vi "test_compressor.vi"() -> ()   [LabVIEW 2010]
panel:
  out "elapsed time":dbl[](array[numeric])
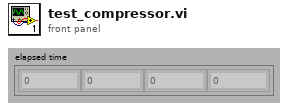
[diagram p1: front panel]
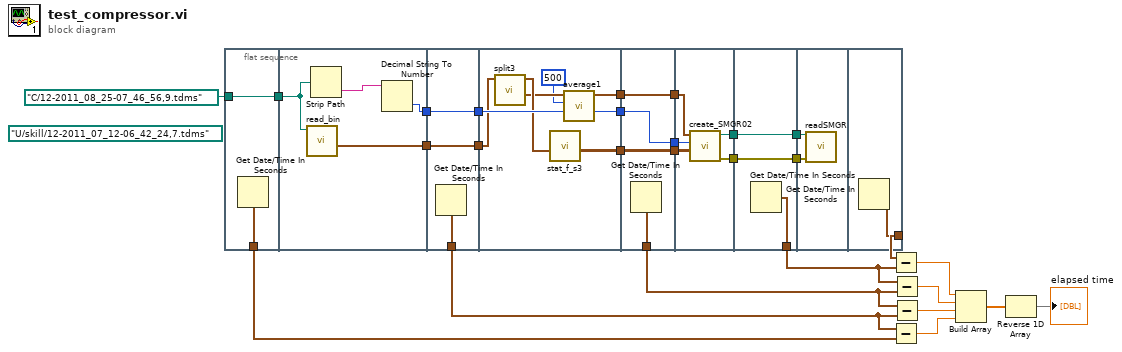
[diagram p0: block diagram]
diagram:
  (unwired) path "U:/skill/12-2011_07_12-06_42_24,7.tdms" ("datalog path (use dialog)")
  n1 = flat-sequence {
    tunnel: path "C:/12-2011_08_25-07_46_56,9.tdms" ("datalog path (use dialog)") -> [w29]
    tunnel: [w29] -> w26
    tunnel: [w28] -> w12
    tunnel: w26 -> [w32]
    tunnel: [w30] -> w24
    tunnel: [w31] -> w17
    tunnel: [w36] -> w25
    tunnel: w24 -> [w36]
    tunnel: w17 -> [w35]
    tunnel: [w35] -> w16
    tunnel: [w34] -> w9
    tunnel: w25 -> [w41]
    tunnel: [w43] -> w23
    tunnel: w16 -> [w42]
    tunnel: [w42] -> w15
    tunnel: [w38] -> w1
    tunnel: w23 -> [w47]
    tunnel: [w47] -> w22
    tunnel: w15 -> [w46]
    tunnel: [w46] -> w14
    tunnel: [w45] -> w10
    tunnel: [w44] -> w2
    tunnel: w1 -> [w44]
    tunnel: w22 -> [w52]
    tunnel: [w51] -> w20
    tunnel: [w50] -> w18
    tunnel: w14 -> [w49]
    tunnel: w2 -> [w48]
    tunnel: [w55] -> w21
    tunnel: w20 -> [w55]
    tunnel: [w54] -> w19
    tunnel: w18 -> [w54]
    tunnel: [w53] -> w11
    tunnel: w21 -> [w57]
    tunnel: w19 -> [w56]
    tunnel: [w58] -> w13
    frame #0 {
      n2 = Get Date/Time In Seconds() -> (seconds since 1Jan1904=w28:timestamp)
    }
    frame #1 {
      n3 = call "read_bin.vi"("datalog path"=w32) -> ("Waveform Graph"=w30:waveform(i16)[])  [unwired: 3 in, 3 out]
      n4 = Strip Path(path=w32) -> (name=w33:string)  [unwired: 1 out]
      n5 = Decimal String To Number(string=w33) -> (number=w31:i32)  [unwired: 2 in, 1 out]
    }
    frame #2 {
      n6 = Get Date/Time In Seconds() -> (seconds since 1Jan1904=w34:timestamp)
    }
    frame #3 {
      n7 = call "split3.vi"("Array of Waveform In"=w41) -> ("Sync"=w39:waveform(i16), "Array of Waveform"=w40:waveform(i16)[])  [unwired: 5 in]
      n8 = call "stat_f_s3.vi"("Array of Wfm"=w40) -> ("Array 2"=w43:waveform(i16)[][])  [unwired: 6 in]
      n9 = call "average1.vi"("Size"=500, "SignalIn"=w39) -> ("output waveform"=w38:waveform(i16))  [unwired: 5 in]
    }
    frame #4 {
      n10 = Get Date/Time In Seconds() -> (seconds since 1Jan1904=w45:timestamp)
    }
    frame #5 {
      n11 = call "create_SMGR02.vi"("array"=w52, "meas_point"=w49, "sync"=w48) -> ("error out"=w50:errorcluster, "original path"=w51:path)  [unwired: 4 in, 1 out]
    }
    frame #6 {
      n12 = Get Date/Time In Seconds() -> (seconds since 1Jan1904=w53:timestamp)
    }
    frame #7 {
      n13 = call "readSMGR.vi"("error in"=w56, "file path"=w57) -> ()  [unwired: 3 in, 3 out]
    }
    frame #8 {
      n14 = Get Date/Time In Seconds() -> (seconds since 1Jan1904=w58:timestamp)
    }
  }
  n15 = Subtract(x=w13, y=w11) -> (x-y=w8:dbl)
  n16 = Subtract(x=w9, y=w12) -> (x-y=w5:dbl)
  n17 = Subtract(x=w11, y=w10) -> (x-y=w7:dbl)
  n18 = Subtract(x=w10, y=w9) -> (x-y=w6:dbl)
  n19 = Build Array(w8, w7, w6, w5) -> (w4:dbl[])
  n20 = Reverse 1D Array(array=w4) -> (reversed array=→"elapsed time":dbl[])
